vi "Get Object Refs from Node.vi"(8 "error in (no error)":errorcluster, 10 "Refresh UI":T1, 11 "Data Value Reference in":T2) -> (0 "error out":errorcluster, 2 "Refresh UI out":T1, 3 "References":T3)   [LabVIEW 2014, in "DAQmx Module Editor Node.lvclass"]
doc: "Gets the reference to the engine and a generic Module Editor Node reference from the node we have. This will be used for operations in the UI."
uses:
  DAQmx Module Editor Node.lvclass
  <vilib>/NI/DCAF/Tag Editor Core/Table API/Table Manager/object ref.ctl
  <vilib>/NI/DCAF/Tag Editor Core/Configuration Editor/Classes/Engine Parent/Engine Parent Editor Node.lvclass
  <vilib>/NI/DCAF/Tag Editor Core/Configuration Editor/Classes/Module editor node/module editor node.lvclass
  <vilib>/NI/Configuration Framework/Node/NodeRef.ctl
  <vilib>/NI/Configuration Framework/Node/NISE_CEF_Node.lvclass
  <vilib>/NI/Configuration Framework/Node/RefreshUIEvent.ctl
  <vilib>/NI/DCAF/Tag Editor Core/Table API/Table Manager/Table Manager.lvclass
  <vilib>/NI/Module Execution Interface/Engine Configuration/engine configuration.lvclass
  <vilib>/NI/Configuration Framework/serializable configuration/NISE_CEF_serializable configuration.lvclass
  testing/DAQmx Module Tests.lvlib
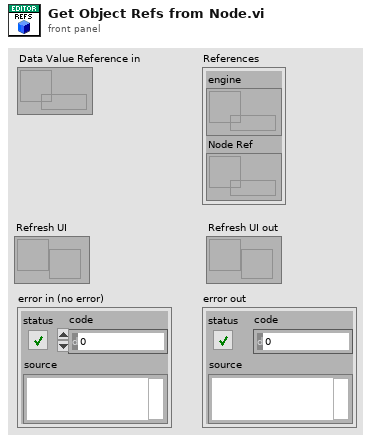
[diagram p1: front panel]
types:
  T1 = typedef "NISE_CEF_Node.lvclass/RefreshUIEvent.ctl" = refnum<user-event>
  T2 = typedef "NISE_CEF_Node.lvclass/NodeRef.ctl" = refnum<data-value>
  T3 = typedef "Table Manager.lvlib/Table Manager.lvclass/object ref.ctl" = cluster{"engine":refnum<data-value>, "Node Ref":refnum<data-value>}
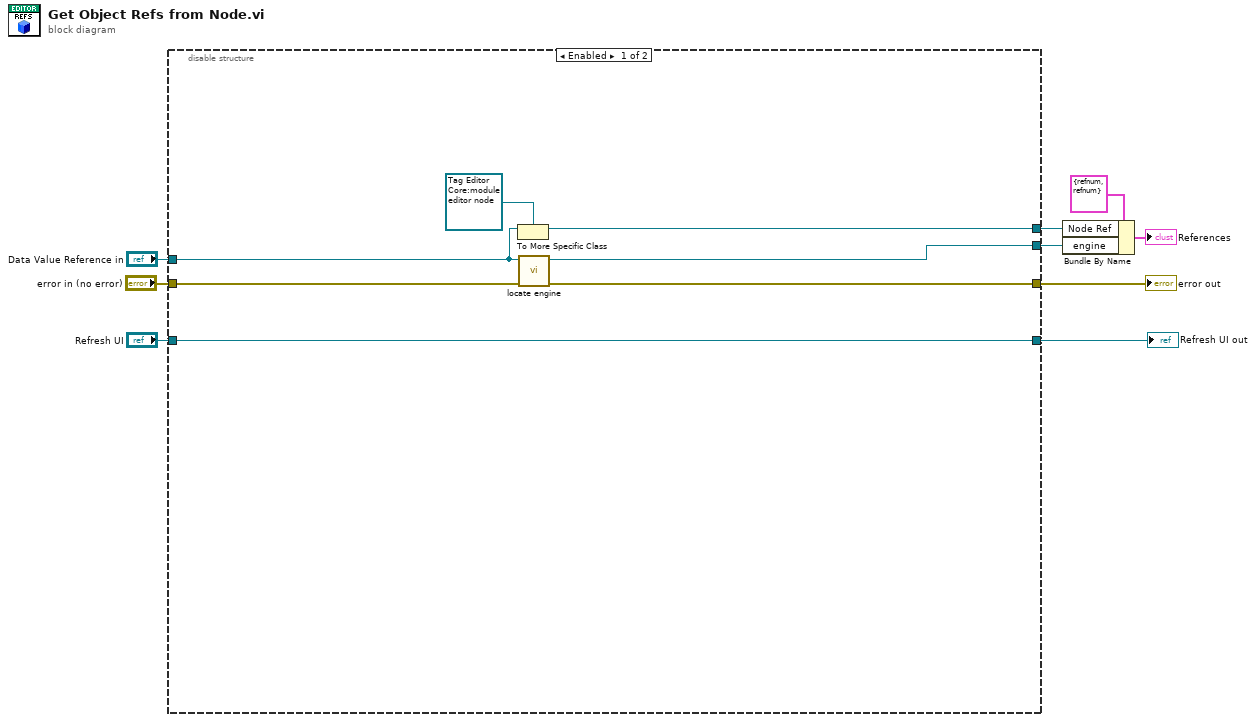
[diagram p0: block diagram]
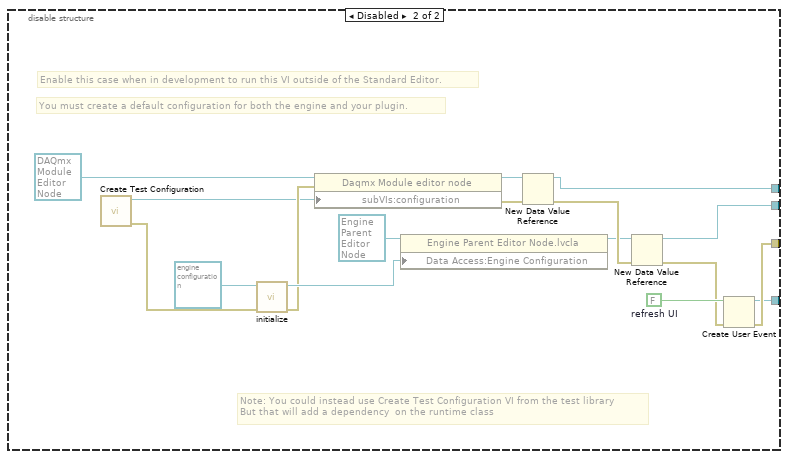
[diagram p2: hidden frame]
diagram:
  n1 = disable-structure shown="Enabled" {
    disable-tunnel: [w16 w23] -> w9
    disable-tunnel: "error in (no error)" -> [w15 _]
    disable-tunnel: [w14 w25] -> w7
    disable-tunnel: "Data Value Reference in" -> [w13 _]
    disable-tunnel: [w11 w24] -> w4
    disable-tunnel: [w10 w22] -> w1
    disable-tunnel: "Refresh UI" -> [w10 _]
    frame Enabled {
      n2 = To More Specific Class(target class=refnum<data-value> refnum ("data value reference"), reference=w13) -> (specific class reference=w14:refnum<data-value>)  [unwired: 1 in, 1 out]
      n3 = call <vilib>:"locate engine.vi"("error in"=w15, "component"=w13) -> ("error out"=w16:errorcluster, "engine"=w11:refnum<data-value>)  [unwired: 8 in]
    }
    frame Disabled {
      w31 = FALSE  # refresh UI
      # "Note: You could instead use Create Test Configuration VI from the test library\nBut that will add a dependency  on the runtime class"
      # "You must create a default configuration for both the engine and your plugin."
      # "Enable this case when in development to run this VI outside of the Standard Editor."
      n4 = call "Create Test Configuration.vi"() -> ("error out"=w17:errorcluster, "Module Configuration"=w18:refnum<class "DAQmx Module Configuration.lvclass">)  [unwired: 6 in, 4 out]
      n5 = call <vilib>:"initialize.vi"("error in"=w17, "configuration in"=refnum<class "engine configuration.lvclass"> refnum ("engine configuration")) -> ("error out"=w19:errorcluster, "configuration out"=w20:refnum<class "engine configuration.lvclass">)  [unwired: 7 in, 1 out]
      n6 = property class="Daqmx Module editor node"(reference=refnum<class "DAQmx Module Editor Node.lvclass"> refnum ("tag bus configurable plugin editor node"), error in=w19, "subVIs:configuration"=w18) -> (reference out=w27:refnum<class "DAQmx Module Editor Node.lvclass">, error out=w33:errorcluster)
      n7 = property class="Engine Parent Editor Node.lvcla"(reference=refnum<class "Engine Parent Editor Node.lvclass"> refnum ("PL Framework Configuration Tool.lvlib:Engine Parent Editor Node.lvclass"), "Data Access:Engine Configuration"=w20) -> (reference out=w28:refnum<class "Engine Parent Editor Node.lvclass">)  [unwired: 1 in, 1 out]
      n8 = New Data Value Reference(data value=w27, error in=w33) -> (data value reference=w25:refnum<data-value>, error out=w32:errorcluster)
      n9 = New Data Value Reference(data value=w28, error in=w32) -> (data value reference=w24:refnum<data-value>, error out=w30:errorcluster)
      n10 = Create User Event(user event datatype=w31, error in=w30) -> (user event=w22:refnum<user-event>, error out=w23:errorcluster)
    }
  }
  "error out" <- w9
  "Refresh UI out" <- w1
  n11 = Bundle By Name(cluster=T3 {"engine"=refnum, "Node Ref"=refnum} ("references"), "Node Ref"=w7, "engine"=w4) -> (→"References":T3)
